vi "Main.vi"() -> ()   [LabVIEW 2017]
doc: "The myRIO Project template acquires acceleration data from the onboard accelerometer and displays the changes of acceleration values in a waveform chart."
panel:
  in  "Stop Button":bool
  in  "String":string
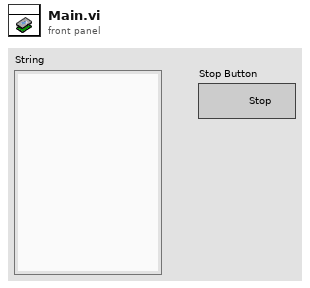
[diagram p1: front panel]
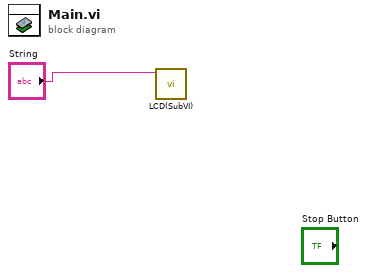
[diagram p0: block diagram]
diagram:
  n1 = call "LCD(SubVI).vi"("String"="String") -> ()  [unwired: 11 in]
